vi "Auto_Routine_StraightTwoPieceCenterMoveCenterLineTRAJ.vi"(8 "error in (no error)":errorcluster) -> (0 "error out":errorcluster)   [LabVIEW 2023]
uses:
  Trajectory/TrajectoryGlobals.vi
  <vilib>/Rock Robotics/WPI/ThirdParty/JAS_Junk/TrajLib/Trajectory_Library.lvlib
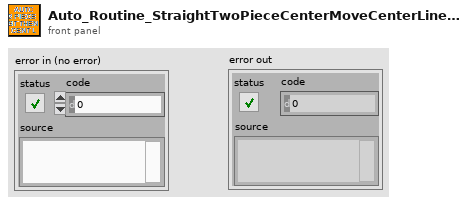
[diagram p1: front panel]
types:
  T1 = typedef "Trajectory_Library.lvlib/TRAJECTORY.ctl" = cluster{"TotalTImeSecs":dbl, "States":T2[]}
  T2 = typedef "Trajectory_Library.lvlib/TRAJ_STATE.ctl" = cluster{"TimeSeconds":dbl, "Velocity":dbl, "Acceleration":dbl, "POSE":T3, "Curvature":dbl}
  T3 = typedef "Trajectory_Library.lvlib/POSE2D.ctl" = cluster{"TRANSLATION":T4, "ROTATION":T5}
  T4 = typedef "Trajectory_Library.lvlib/TRANSLATION2D.ctl" = cluster{"X":dbl, "Y":dbl}
  T5 = typedef "Trajectory_Library.lvlib/ROTATION2D.ctl" = cluster{"VALUE":dbl, "COS":dbl, "SIN":dbl}
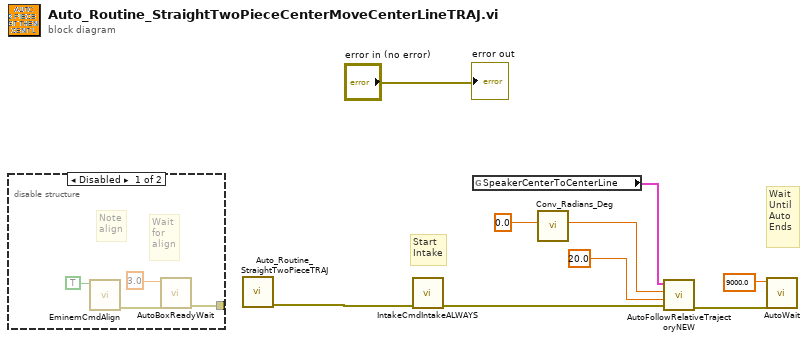
[diagram p0: block diagram]
diagram:
  # "Start\nIntake"
  # "Wait\nUntil\nAuto \nEnds"
  n1 = disable-structure shown="Disabled" {
    disable-tunnel: [w10 _] -> _
    frame Disabled {
      # "Wait\nfor\nalign"
      # "Note\nalign"
      n2 = call "EminemCmdAlign.vi"("box align"=TRUE) -> ("error out"=w11:errorcluster)  [unwired: 10 in]
      n3 = call "AutoBoxReadyWait.vi"("error in (no error)"=w11, "TimeOut (s)"=3.0) -> ("error out"=w10:errorcluster)  [unwired: 9 in]
    }
    frame Enabled {
    }
  }
  n4 = call "Auto_Routine_StraightTwoPieceTRAJ.vi"() -> ("error out"=w2:errorcluster)  [unwired: 11 in]
  n5 = call "IntakeCmdIntakeALWAYS.vi"("error in (no error)"=w2) -> ("error out"=w1:errorcluster)  [unwired: 10 in]
  n6 = global read "TrajectoryGlobals.vi" "SpeakerCenterToCenterLine"() -> (w7:T1)
  n7 = call <vilib>:"Conv_Radians_Deg.vi"("Radians"=0.0) -> ("Degrees"=w5:dbl)  [unwired: 10 in]
  n8 = call "AutoFollowRelativeTrajectoryNEW.vi"("error in (no error)"=w1, "TimeOut (s)"=20.0, "End Orientation"=w5, "Trajectory"=w7) -> ("error out"=w3:errorcluster)  [unwired: 7 in]
  n9 = call "AutoWait.vi"("error in (no error)"=w3, "TimeOut (s)"=9000.0) -> ()  [unwired: 9 in, 1 out]
  "error out" <- "error in (no error)"
